vi "Read Multiple Measurements (Current Data).vi"(0 "VISA resource name":refnum<visa-resource-name>, 5 "Maximum Time (30000 ms)":i32=30000, 11 "error in (no error)":errorcluster) -> (4 "VISA resource name out":refnum<visa-resource-name>, 6 "Instantaneous Current":dbl[](array[numeric]), 8 "Current Harmonic Amplitudes":dbl[](array[numeric]), 10 "Current Harmonic Phase Angles":dbl[](array[numeric]), 15 "error out":errorcluster)   [LabVIEW 2020, in "Agilent 681x Series.lvlib"]
doc: "Initiates and reads 4096 instantaneous current measurements, the first 50 current harmonic amplitudes and phase values.\n\n<B>Note:</B>\n\nThis VI changes the <B>Trigger Source</B> to <B>Bus</B> and uses a software trigger after the instrument is initiated. If you want to control the triggering and other features, please use the low level VIs."
uses:
  <instrlib>/Agilent 681x Series/Agilent 681x Series.lvlib
  <instrlib>/Agilent 681x Series/Public/Data/Low Level/Fetch Multiple Measurements (Current Data).vi
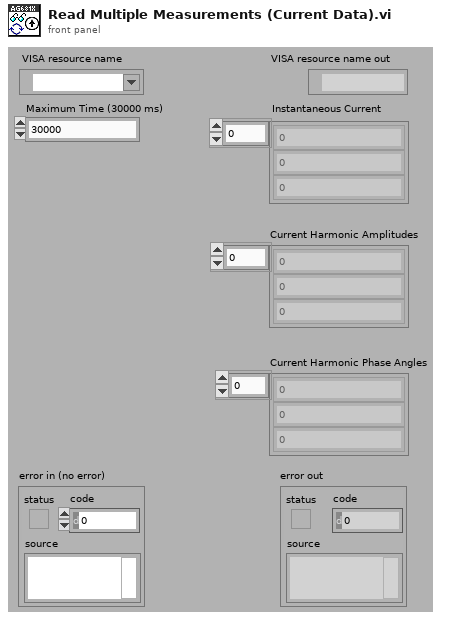
[diagram p1: front panel]
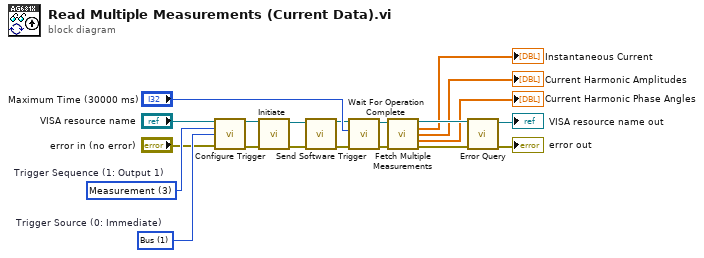
[diagram p0: block diagram]
diagram:
  w9 = 1 items=["Immediate", "Bus", "External", "Phase", "Trigger Out"]  # Trigger Source (0: Immediate)
  w10 = 3 items=["Output"=1, "Synchronous Source"=2, "Measurement"=3]  # Trigger Sequence (1: Output 1)
  n1 = call <instrlib>:"Configure Trigger.vi"("VISA resource name"="VISA resource name", "Trigger Sequence (1: Output 1)"=w10, "Trigger Source (0: Immediate)"=w9, "error in (no error)"="error in (no error)") -> ("VISA resource name out"=w7:refnum<visa-resource-name>, "error out"=w8:errorcluster)  [unwired: 10 in]
  n2 = call <instrlib>:"Initiate.vi"("error in (no error)"=w8, "VISA resource name"=w7) -> ("error out"=w6:errorcluster, "VISA resource name out"=w5:refnum<visa-resource-name>)  [unwired: 8 in]
  n3 = call <instrlib>:"Send Software Trigger.vi"("VISA resource name"=w5, "error in (no error)"=w6) -> ("VISA resource name out"=w4:refnum<visa-resource-name>, "error out"=w3:errorcluster)  [unwired: 12 in]
  n4 = call <instrlib>:"Wait For Operation Complete.vi"("error in (no error)"=w3, "Maximum Time (10000 ms)"="Maximum Time (30000 ms)", "VISA resource name"=w4) -> ("error out"=w17:errorcluster, "VISA resource name out"=w16:refnum<visa-resource-name>)  [unwired: 7 in]
  n5 = call-poly <instrlib>:"Fetch Multiple Measurements.vi"("VISA resource name"=w16, "error in (no error)"=w17) -> ("VISA resource name out"=w15:refnum<visa-resource-name>, "Instantaneous Current"=→"Instantaneous Current":dbl[], "Current Harmonic Amplitudes"=→"Current Harmonic Amplitudes":dbl[], "Current Harmonic Phase Angles"=→"Current Harmonic Phase Angles":dbl[], "error out"=w14:errorcluster)  [unwired: 9 in]
  n6 = call <instrlib>:"Error Query.vi"("error in (no error)"=w14, "VISA resource name"=w15) -> ("error out"=→"error out":errorcluster, "VISA resource name out"=→"VISA resource name out":refnum<visa-resource-name>)  [unwired: 6 in, 2 out]
